vi "Motion_Loader Enable.vi"(8 "error in (no error)":errorcluster, 10 "Enable? (T)":bool=TRUE, 11 "TCP Connection Refnum in":refnum<k5>) -> (0 "error out":errorcluster, 3 "TCP Connection Refnum (dup)":refnum<k5>)   [LabVIEW 2010]
uses:
  Motion_Coils Typedef.ctl
  <vilib>/NI Modbus.llb/MB Ethernet Master Query Write Single Coil (poly).vi
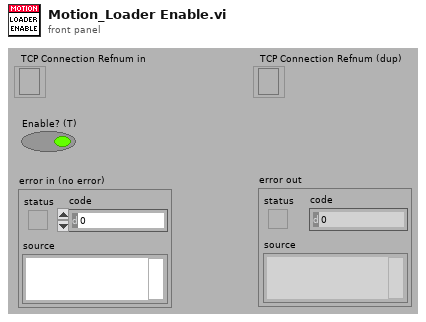
[diagram p1: front panel]
types:
  T1 = typedef "Motion_Coils Typedef.ctl" = u16
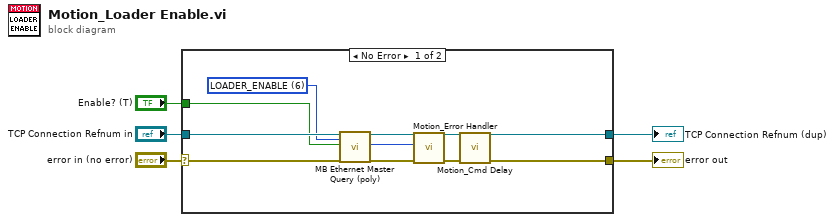
[diagram p0: block diagram]
diagram:
  n1 = case shown="No Error" "error in (no error)" {
    selector: "error in (no error)" -> [w16 w18]
    tunnel: [w8 w18] -> w4
    tunnel: "TCP Connection Refnum in" -> [w15 w17]
    tunnel: [w10 w17] -> w2
    tunnel: "Enable? (T)" -> [w6 _]
    frame No Error {
      w14 = T1 6 items=["GANTRY_ALARM_CLEAR", "GANTRY_ENABLE", "GANTRY_HOME", "GANTRY_GOTO", "LOADER_HOME", "LOADER_ALARM_CLEAR", "LOADER_ENABLE", "LOADER_GOTO_CONNECT", "LOADER_GOTO_LOAD", "LOADER_STOP"] ("Coils")
      n2 = call-poly <vilib>:"MB Ethernet Master Query (poly).vi"("TCP Connection Refnum in"=w15, "Address"=w14, "Coil"=w6, "error in"=w16) -> ("TCP Connection Refnum (dup)"=w12:refnum<k5>, "Exception Code"=w11:u8, "error out"=w13:errorcluster)  [unwired: 13 in]
      n3 = call "Motion_Error Handler.vi"("error in (no error)"=w13, "Exception Code"=w11, "TCP Connection Refnum in"=w12) -> ("error out"=w7:errorcluster, "TCP Connection Refnum (dup)"=w9:refnum<k5>)  [unwired: 7 in]
      n4 = call "Motion_Cmd Delay.vi"("error in"=w7, "TCP Connection Refnum"=w9) -> ("error out"=w8:errorcluster, "TCP Connection Refnum (dup)"=w10:refnum<k5>)  [unwired: 8 in]
    }
    frame Error {
    }
  }
  "error out" <- w4
  "TCP Connection Refnum (dup)" <- w2
